vi "Notch Filter Coefficients.vi"(8 "harmonics":i32, 9 "Q":dbl, 10 "notch (Hz)":dbl, 11 "Sample rate (Hz)":dbl) -> (1 "Forward Coefficients":dbl[](array[numeric]), 2 "Reverse Coefficients":dbl[](array[numeric]), 3 "IIR Filter Cluster":T1)   [LabVIEW 2019, in "DSP.lvclass"]
uses:
  DSP.lvclass
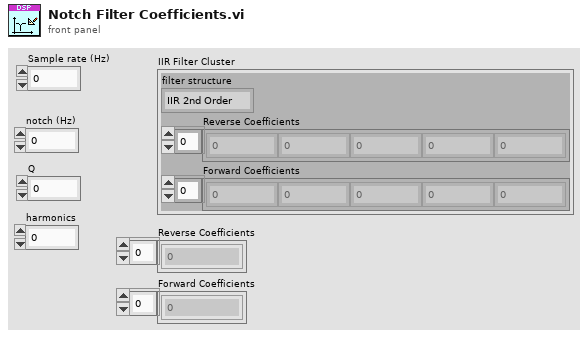
[diagram p1: front panel]
types:
  T1 = cluster{"filter structure":enum32{"IIR 2nd Order", "IIR 4th Order"}, "Reverse Coefficients":dbl[], "Forward Coefficients":dbl[]}
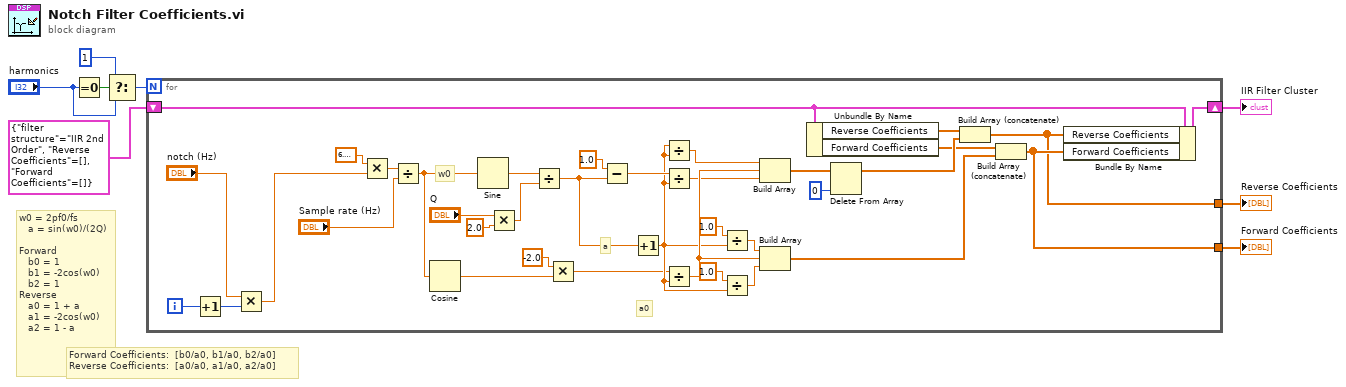
[diagram p0: block diagram]
diagram:
  # "Forward Coefficients:  [b0/a0, b1/a0, b2/a0]\nReverse Coefficients:  [a0/a0, a1/a0, a2/a0]"
  # "w0 = 2pf0/fs\n   a = sin(w0)/(2Q)\n   \nForward\n   b0 = 1\n   b1 = -2cos(w0)\n   b2 = 1\nReverse\n   a0 = 1 + a\n   a1 = -2cos(w0)\n   a2 = 1 - a"
  n1 = Equal To 0?(x="harmonics") -> (x = 0?=w8:bool)
  n2 = Select(t=1, s=w8, f="harmonics") -> (s? t:f=w6:i32)
  n3 = for {
    N: w6 -> [_]
    shift-right: [w13] -> w3
    shift-left: T1 {"filter structure"=enum."IIR 2nd Order", "Reverse Coefficients"=[], "Forward Coefficients"=[]} ("IIR Filter Cluster") -> [w14]
    tunnel: [w10] -> w2
    tunnel: [w9] -> w1
    i -> [w20]
    # "a0"
    # "a"
    # "w0"
    n4 = Increment(x=w20) -> (x+1=w19:i32)
    n5 = Multiply(x="notch (Hz)", y=w19) -> (x*y=w18:dbl)
    n6 = Multiply(x=6.283185307179586, y=w18) -> (x*y=w24:dbl)
    n7 = Divide(x=w24, y="Sample rate (Hz)") -> (x/y=w34:dbl)
    n8 = Cosine(x=w34) -> (cos(x)=w33:dbl)
    n9 = Sine(x=w34) -> (sin(x)=w26:dbl)
    n10 = Multiply(x="Q", y=2.0) -> (x*y=w29:dbl)
    n11 = Divide(x=w26, y=w29) -> (x/y=w43:dbl)
    n12 = Multiply(x=-2.0, y=w33) -> (x*y=w35:dbl)
    n13 = Subtract(x=1.0, y=w43) -> (x-y=w44:dbl)
    n14 = Increment(x=w43) -> (x+1=w39:dbl)
    n15 = Divide(x=w39, y=w39) -> (x/y=w38:dbl)
    n16 = Divide(x=w44, y=w39) -> (x/y=w40:dbl)
    n17 = Divide(x=w35, y=w39) -> (x/y=w41:dbl)
    n18 = Divide(x=1.0, y=w39) -> (x/y=w30:dbl)
    n19 = Divide(x=1.0, y=w39) -> (x/y=w37:dbl)
    n20 = Build Array(w38, w41, w40) -> (w22:dbl[])
    n21 = Build Array(w30, w41, w37) -> (w11:dbl[])
    n22 = Unbundle By Name(w14) -> ("Reverse Coefficients"=w12:dbl[], "Forward Coefficients"=w15:dbl[])
    n23 = Delete From Array(array=w22, index=0) -> (array with subset deleted=w16:dbl[])  [unwired: 1 in, 1 out]
    n24 = Build Array (concatenate)(w12, w16) -> (w9:dbl[])
    n25 = Build Array (concatenate)(w15, w11) -> (w10:dbl[])
    n26 = Bundle By Name(cluster=w14, "Reverse Coefficients"=w9, "Forward Coefficients"=w10) -> (w13:T1)
  }
  "IIR Filter Cluster" <- w3
  "Reverse Coefficients" <- w1
  "Forward Coefficients" <- w2
